vi "IDS_SubMasterExample_ErrorMessages.vi"(3 "String in 1":refnum<vi>, 4 "String in 2":refnum<vi>, 5 "String in 3":refnum<vi>, 11 "appended array":errorcluster[](array[cluster])) -> ()   [LabVIEW 2016]
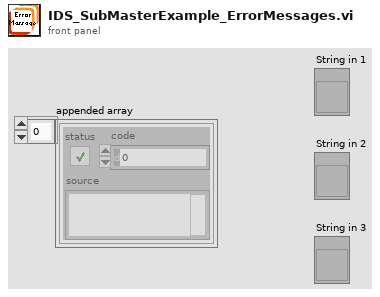
[diagram p1: front panel]
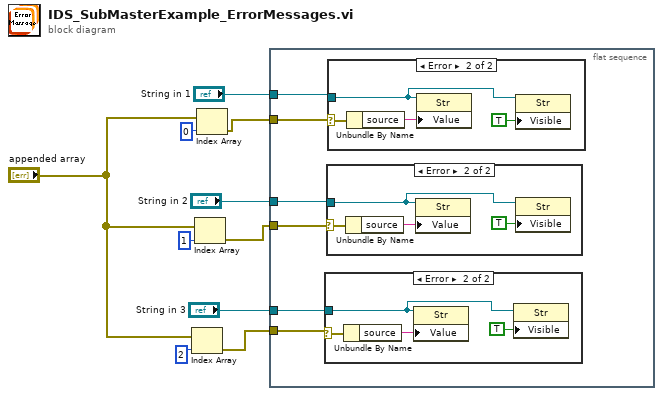
[diagram p0: block diagram]
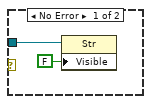
[diagram p2: hidden frame]
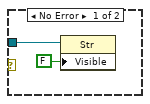
[diagram p3: hidden frame]
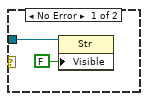
[diagram p4: hidden frame]
diagram:
  n1 = Index Array(array="appended array", index=2) -> (element=w3:errorcluster)
  n2 = Index Array(array="appended array", index=1) -> (element=w5:errorcluster)
  n3 = Index Array(array="appended array", index=0) -> (element=w6:errorcluster)
  n4 = flat-sequence {
    tunnel: "String in 1" -> [w16]
    tunnel: "String in 2" -> [w15]
    tunnel: "String in 3" -> [w14]
    tunnel: w6 -> [w13]
    tunnel: w5 -> [w12]
    tunnel: w3 -> [w11]
    frame #0 {
      n5 = case shown="Error" w11 {
        selector: w11 -> [_ w21]
        tunnel: w14 -> [w18 w19]
        frame No Error {
          n6 = property class="Str"(reference=w18, "Visible"=FALSE) -> ()  [unwired: 1 in, 2 out]
        }
        frame Error {
          n7 = Unbundle By Name(w21) -> ("source"=w22:string)
          n8 = property class="Str"(reference=w19, "Value"=w22) -> ()  [unwired: 1 in, 2 out]
          n9 = property class="Str"(reference=w19, "Visible"=TRUE) -> ()  [unwired: 1 in, 2 out]
        }
      }
      n10 = case shown="Error" w12 {
        selector: w12 -> [_ w27]
        tunnel: w15 -> [w24 w25]
        frame No Error {
          n11 = property class="Str"(reference=w24, "Visible"=FALSE) -> ()  [unwired: 1 in, 2 out]
        }
        frame Error {
          n12 = Unbundle By Name(w27) -> ("source"=w28:string)
          n13 = property class="Str"(reference=w25, "Value"=w28) -> ()  [unwired: 1 in, 2 out]
          n14 = property class="Str"(reference=w25, "Visible"=TRUE) -> ()  [unwired: 1 in, 2 out]
        }
      }
      n15 = case shown="Error" w13 {
        selector: w13 -> [_ w33]
        tunnel: w16 -> [w30 w31]
        frame No Error {
          n16 = property class="Str"(reference=w30, "Visible"=FALSE) -> ()  [unwired: 1 in, 2 out]
        }
        frame Error {
          n17 = Unbundle By Name(w33) -> ("source"=w34:string)
          n18 = property class="Str"(reference=w31, "Value"=w34) -> ()  [unwired: 1 in, 2 out]
          n19 = property class="Str"(reference=w31, "Visible"=TRUE) -> ()  [unwired: 1 in, 2 out]
        }
      }
    }
  }
